vi "solar_voy_def Import (cmd_tlm_server).vi"(6 "Suppress Errors? (T)":bool=TRUE, 8 "error in (no error)":errorcluster, 11 "cmd_tlm_server.txt":path) -> (0 "error out":errorcluster, 3 "INTERFACES":T1[](array[typedef]))   [LabVIEW 2018]
doc: "This imports a COSMOS command and telemetry server file. Refer to http://cosmosrb.com/docs/interfaces/"
uses:
  solar_voy_def_ctl INTERFACE.ctl
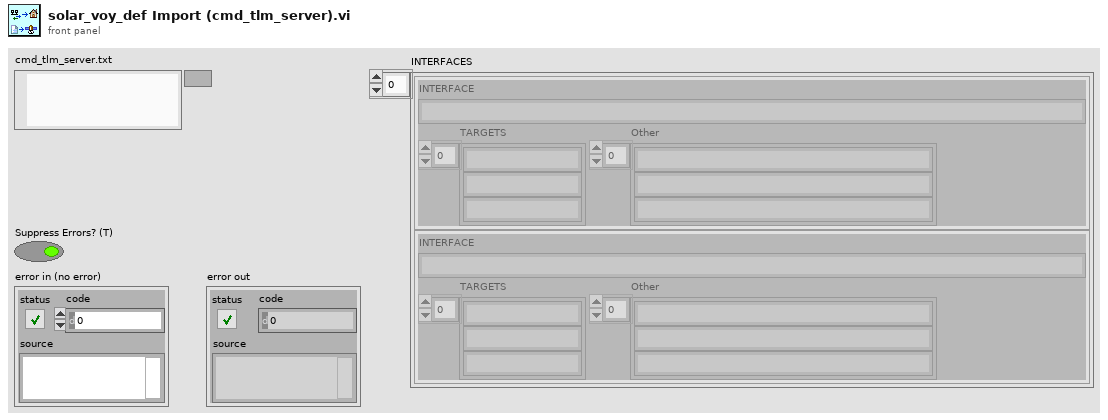
[diagram p1: front panel]
types:
  T1 = typedef "solar_voy_def_ctl INTERFACE.ctl" = cluster{"INTERFACE":string, "TARGETS":string[], "Other":string[]}
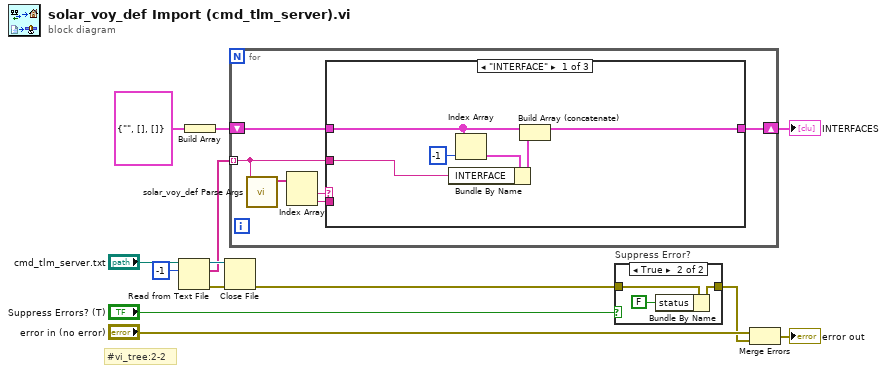
[diagram p0: block diagram]
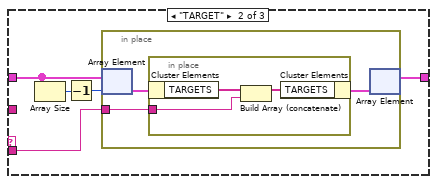
[diagram p2: hidden frame]
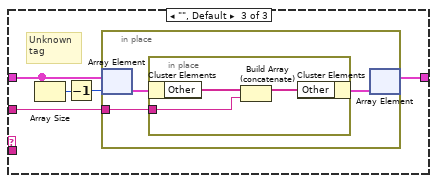
[diagram p3: hidden frame]
diagram:
  # "#vi_tree:2-2"
  n1 = Read from Text File(file (use dialog)="cmd_tlm_server.txt", count=-1) -> (refnum out=w7:refnum<file>, text=w5:string[], error out=w6:errorcluster)  [unwired: 2 in, 1 out]
  n2 = Build Array(T1 {"INTERFACE"="", "TARGETS"=[], "Other"=[]} ("INTERFACE")) -> (w4:T1[])
  n3 = Close File(refnum=w7, error in=w6) -> (error out=w2:errorcluster)  [unwired: 1 out]
  n4 = for {
    tunnel: w5 -> [w14] mode=indexing
    shift-right: [w18] -> w3
    shift-left: w4 -> [w19]
    n5 = call "solar_voy_def Parse Args.vi"("String"=w14) -> ("Arguments"=w16:string[])  [unwired: 10 in]
    n6 = Index Array(array=w16) -> (element #1=w17:string, element #2=w15:string)  [unwired: 2 in]
    n7 = case shown="\"INTERFACE\"" w17 {
      tunnel: w19 -> [w24 w30 w41]
      tunnel: [w25 w27 w38] -> w18
      tunnel: w15 -> [_ w26 _]
      tunnel: w14 -> [w20 _ w37]
      frame "INTERFACE" {
        n8 = Index Array(array=w24, index=-1) -> (element=w22:T1)
        n9 = Bundle By Name(cluster=w22, "INTERFACE"=w20) -> (w21:T1)
        n10 = Build Array (concatenate)(w24, w21) -> (w25:T1[])
      }
      frame "TARGET" {
        n11 = Array Size(array=w30) -> (size(s)=w29:i32)
        n12 = Decrement(x=w29) -> (x-1=w28:i32)
        n13 = in-place {
          in-place-border: w26 -> [w32]
          n14 = in-place-array #1(w30, w28) -> (w33:T1)
          n15 = in-place {
            in-place-border: w32 -> [w34]
            n16 = in-place-cluster #2(w33) -> ("TARGETS"=w36:string[])
            n17 = Build Array (concatenate)(w36, w34) -> (w35:string[])
            n18 = in-place-cluster #2("TARGETS"=w35) -> (w31:T1)
          }
          n19 = in-place-array #1(w31) -> (w27:T1[])  [unwired: 1 out]
        }
      }
      frame "", Default {
        # "Unknown\ntag"
        n20 = Array Size(array=w41) -> (size(s)=w40:i32)
        n21 = Decrement(x=w40) -> (x-1=w39:i32)
        n22 = in-place {
          in-place-border: w37 -> [w43]
          n23 = in-place-array #3(w41, w39) -> (w44:T1)
          n24 = in-place {
            in-place-border: w43 -> [w45]
            n25 = in-place-cluster #4(w44) -> ("Other"=w47:string[])
            n26 = Build Array (concatenate)(w47, w45) -> (w46:string[])
            n27 = in-place-cluster #4("Other"=w46) -> (w42:T1)
          }
          n28 = in-place-array #3(w42) -> (w38:T1[])  [unwired: 1 out]
        }
      }
    }
  }
  "INTERFACES" <- w3
  n29 = case "Suppress Error?" shown="True" "Suppress Errors? (T)" {
    tunnel: w2 -> [w48 w51]
    tunnel: [w48 w50] -> w11
    frame False {
    }
    frame True {
      n30 = Bundle By Name(cluster=w51, "status"=FALSE) -> (w50:errorcluster)
    }
  }
  n31 = Merge Errors("error in (no error)", w11) -> (→"error out":errorcluster)
